vi "Generate Local Event.vi"(8 "error in (no error)":errorcluster, 10 "Data":variant, 11 "Event Type":T1=enum."Button 0 Click") -> (0 "error out":errorcluster)   [LabVIEW 2019, in "FootScan Engine.lvlib"]
uses:
  FootScan Engine.lvlib
  Event/Event Type.ctl
  Event/FootScan Engine Event.lvlib
panel:
  # "Input"
  # "Output"
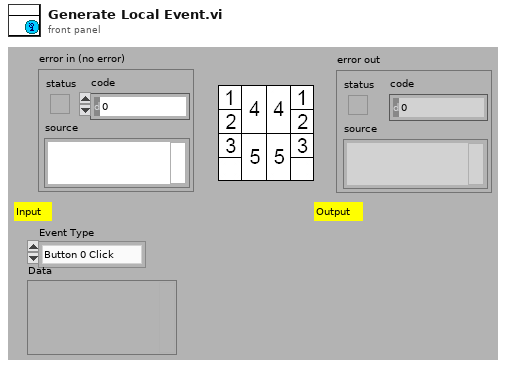
[diagram p1: front panel]
types:
  T1 = typedef "FootScan Engine Event.lvlib/Event Type.ctl" = enum16{"Default", "Initialize Finish", "Button 0 Click", "Exit Click", "Exit"}
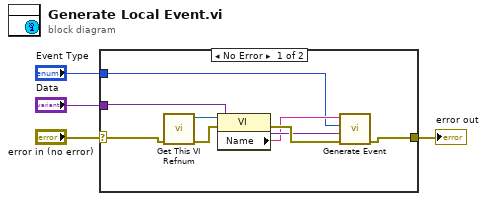
[diagram p0: block diagram]
diagram:
  n1 = case shown="No Error" "error in (no error)" {
    selector: "error in (no error)" -> [w12 w13]
    tunnel: [w5 w13] -> w3
    tunnel: "Data" -> [w8 _]
    tunnel: "Event Type" -> [w6 _]
    frame No Error {
      n2 = call "Get This VI Refnum.vi"("error in (no error)"=w12) -> ("error out"=w10:errorcluster, "This VI Refnum Out"=w11:refnum<vi>)  [unwired: 9 in]
      n3 = property class="VI"(reference=w11, error in=w10) -> (error out=w9:errorcluster, "Name"=w7:string)  [unwired: 1 out]
      n4 = call "Generate Event.vi"("error in (no error)"=w9, "Data"=w8, "Event Type"=w6, "Sender"=w7) -> ("error out"=w5:errorcluster)  [unwired: 7 in]
    }
    frame Error {
    }
  }
  "error out" <- w3
